vi "Downsample Image.vi"(8 "error in":errorcluster, 10 "Reduction Factor":i32, 11 "Refnum in":T1) -> (0 "error out":errorcluster, 3 "Refnum out":T1)   [LabVIEW 2022 SP3]
uses:
  <vilib>/vision/Image Controls.llb/IMAQ Image.ctl
  Vision/Vision.lvlib
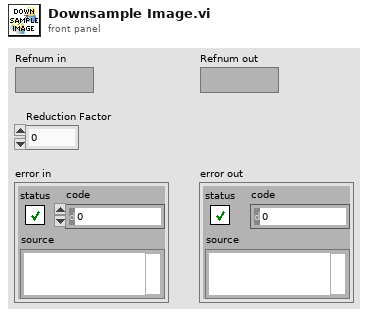
[diagram p1: front panel]
types:
  T1 = typedef "IMAQ Image.ctl" = refnum<image>
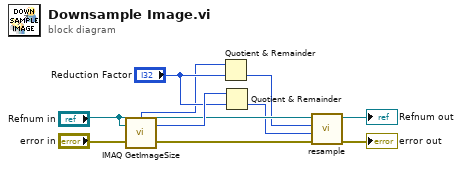
[diagram p0: block diagram]
diagram:
  n1 = call "IMAQ GetImageSize"("Image"="Refnum in", "error in (no error)"="error in") -> ("Y Resolution"=w10:i32, "X Resolution"=w8:i32, "error out"=w6:errorcluster)  [unwired: 2 in]
  n2 = Quotient & Remainder(x=w8, y="Reduction Factor") -> (floor(x/y)=w1:i32)  [unwired: 1 out]
  n3 = Quotient & Remainder(x=w10, y="Reduction Factor") -> (floor(x/y)=w2:i32)  [unwired: 1 out]
  n4 = call "resample.vi"("error in (no error)"=w6, "Height"=w2, "Width"=w1, "Image in"="Refnum in") -> ("error out"=→"error out":errorcluster, "Image out"=→"Refnum out":T1)  [unwired: 6 in]
